vi "Teleop.vi"(10 "Match Info":T1={"Autonomous Elapsed Seconds"=0.0, "TeleOp Elapsed Seconds"=0.0, "Disabled Elapsed Seconds"=0.0, "Visited Autonomous"=FALSE, "Visited TeleOp"=FALSE, "Visited Disabled"=FALSE, "Autonomous Settings"={"Autonomous Style"=enum."Independent", "VI Refnum"=refnum}}, 11 "Call Context":T2) -> ()   [LabVIEW 2020]
doc: "This VI is called for each enabled TeleOp packet received from the DS. It is typically used to read from joysticks and other inputs and update I/O or setpoints for timed control loops. It should complete and return within 20 milliseconds or risk missing DS packets."
uses:
  <vilib>/Rock Robotics/WPI/DriverStation/WPI_DriverStationDerivedRobotMode.ctl
  <vilib>/Rock Robotics/WPI/DriverStation/WPI_DriverStationMatch Info.ctl
  <vilib>/Rock Robotics/WPI/Utilities/WPI_GetSetVariantRefNum.vi
  <vilib>/Rock Robotics/Network Tables/NT Write Boolean Array.vi
  Framework/Robot Global Data.vi
  <vilib>/Rock Robotics/Network Tables/NT Write Variant.vi
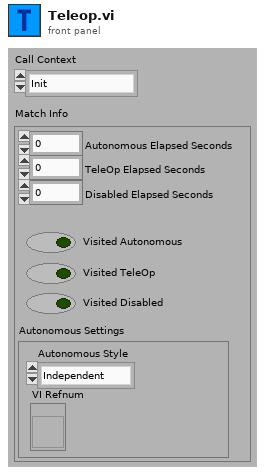
[diagram p1: front panel]
types:
  T1 = typedef "WPI_DriverStationMatch Info.ctl" = cluster{"Autonomous Elapsed Seconds":dbl, "TeleOp Elapsed Seconds":dbl, "Disabled Elapsed Seconds":dbl, "Visited Autonomous":bool, "Visited TeleOp":bool, "Visited Disabled":bool, "Autonomous Settings":cluster{"Autonomous Style":enum16{"Iterative", "Independent"}, "VI Refnum":refnum<vi>}}
  T2 = typedef "WPI_DriverStationDerivedRobotMode.ctl" = enum16{"Init", "Execute", "Stop"}
  T3 = typedef "WPI_JoystickDevRef.ctl" = cluster{"Device":T4}
  T4 = typedef "WPI_JoystickDeviceEnum.ctl" = enum16{"USB 0", "USB 1", "USB 2", "USB 3", "USB 4", "USB 5"}
  T5 = typedef "Command Status Info.ctl" = cluster{"Name":string, "Status":T6, "notifier out":T7}
  T6 = typedef "Completion Status.ctl" = enum16{"Successful", "Aborted", "Incomplete"}
  T7 = typedef "Completion Notifier.ctl" = refnum<notifier>
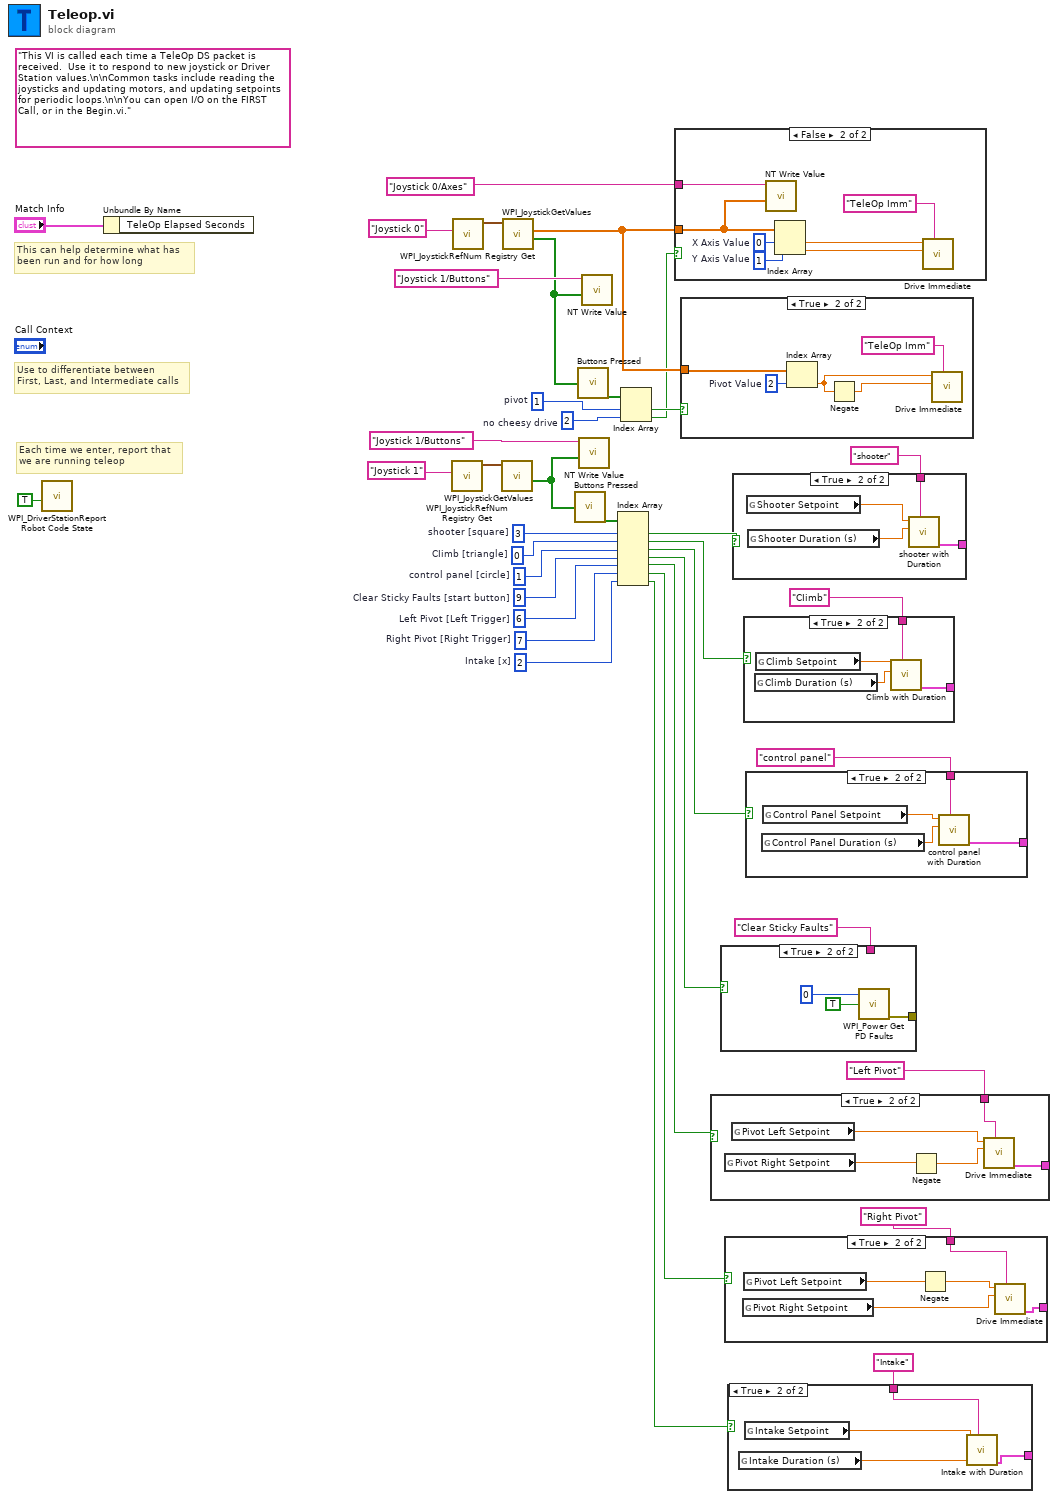
[diagram p0: block diagram]
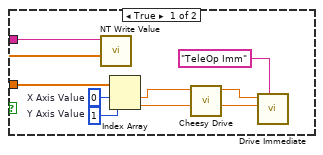
[diagram p2: hidden frame]
diagram:
  w2 = 2  # no cheesy drive
  w7 = 1  # pivot
  w14 = 2  # Intake [x]
  w19 = 7  # Right Pivot [Right Trigger]
  w15 = 6  # Left Pivot [Left Trigger]
  w16 = 9  # Clear Sticky Faults [start button]
  w24 = 1  # control panel [circle]
  w25 = 0  # CIimb [triangle]
  w26 = 3  # shooter [square]
  (unwired) "This VI is called each time a TeleOp DS packet is received.  Use it to respond to new joystick or Driver Station values.\n\nCommon tasks include reading the joysticks and updating motors, and updating setpoints for periodic loops.\n\nYou can open I/O on the FIRST Call, or in the Begin.vi."
  # "Each time we enter, report that\nwe are running teleop"
  # "Use to differentiate between\nFirst, Last, and Intermediate calls"
  # "This can help determine what has\nbeen run and for how long"
  n1 = call <vilib>:"WPI_DriverStationReport Robot Code State.vi"("TeleOp"=TRUE ("Autonomous")) -> ()  [unwired: 10 in, 1 out]
  n2 = Unbundle By Name("Match Info") -> ()  [unwired: 1 out]
  n3 = call <vilib>:"WPI_JoystickRefNum Registry Get.vi"("refnum name"="Joystick 1") -> ("JoystickDevRef"=w11:T3)  [unwired: 1 in, 9 out]
  n4 = call <vilib>:"WPI_JoystickRefNum Registry Get.vi"("refnum name"="Joystick 0") -> ("JoystickDevRef"=w36:T3)  [unwired: 1 in, 9 out]
  n5 = call <vilib>:"WPI_JoystickGetValues.vi"("JoystickDevRef"=w11) -> ("Buttons"=w9:bool[])  [unwired: 6 in, 4 out]
  n6 = call <vilib>:"WPI_JoystickGetValues.vi"("JoystickDevRef"=w36) -> ("Buttons"=w4:bool[], "Axes"=w8:dbl[])  [unwired: 6 in, 3 out]
  n7 = call "Buttons Pressed.vi"("Button Values"=w9) -> ("Button Presses"=w33:bool[])
  n8 = call "Buttons Pressed.vi"("Button Values"=w4) -> ("Button Presses"=w5:bool[])
  n9 = call-poly <vilib>:"NT Write Value.vi"("Boolean Array"=w9, "Name"="Joystick 1/Buttons") -> ()  [unwired: 9 in, 1 out]
  n10 = call-poly <vilib>:"NT Write Value.vi"("Boolean Array"=w4, "Name"="Joystick 1/Buttons") -> ()  [unwired: 9 in, 1 out]
  n11 = Index Array(array=w33, index #1=w26, index #2=w25, index #3=w24, index #4=w16, index #5=w15, index #6=w19, index #7=w14) -> (element #1=w32:bool, element #2=w31:bool, element #3=w27:bool, element #4=w22:bool, element #5=w18:bool, element #6=w17:bool, element #7=w12:bool)
  n12 = Index Array(array=w5, index #1=w7, index #2=w2) -> (element #1=w3:bool, element #2=w1:bool)
  n13 = case shown="False" w1 {
    tunnel: "Joystick 0/Axes" ("Name") -> [w44 w53]
    tunnel: w8 -> [w40 w49]
    frame True {
      w42 = 1  # Y Axis Value
      w43 = 0  # X Axis Value
      n14 = call-poly <vilib>:"NT Write Value.vi"("Variant"=w40, "Name"=w44) -> ()  [unwired: 9 in, 1 out]
      n15 = Index Array(array=w40, index #1=w43, index #2=w42) -> (element #1=w41:dbl, element #2=w45:dbl)
      n16 = call "Cheesy Drive.vi"("Throttle"=w45, "Wheel"=w41) -> ("Right PWM"=w46:dbl, "Left PWM"=w47:dbl)  [unwired: 8 in]
      n17 = call "Drive Immediate.vi"("Description"="TeleOp Imm", "Right Setpoint"=w46, "Left Setpoint"=w47) -> ()  [unwired: 8 in, 1 out]
    }
    frame False {
      w51 = 1  # Y Axis Value
      w52 = 0  # X Axis Value
      n18 = call-poly <vilib>:"NT Write Value.vi"("Variant"=w49, "Name"=w53) -> ()  [unwired: 9 in, 1 out]
      n19 = Index Array(array=w49, index #1=w52, index #2=w51) -> (element #1=w50:dbl, element #2=w54:dbl)
      n20 = call "Drive Immediate.vi"("Description"="TeleOp Imm", "Right Setpoint"=w54, "Left Setpoint"=w50) -> ()  [unwired: 8 in, 1 out]
    }
  }
  n21 = case shown="True" w3 {
    tunnel: w8 -> [_ w58]
    frame False {
    }
    frame True {
      w60 = 2  # Pivot Value
      n22 = Index Array(array=w58, index=w60) -> (element=w57:dbl)
      n23 = Negate(x=w57) -> (-x=w56:dbl)
      n24 = call "Drive Immediate.vi"("Description"="TeleOp Imm", "Right Setpoint"=w56, "Left Setpoint"=w57) -> ()  [unwired: 8 in, 1 out]
    }
  }
  n25 = case shown="True" w18 {
    tunnel: [_ w65] -> _
    tunnel: "Left Pivot" ("Description") -> [_ w64]
    frame False {
    }
    frame True {
      n26 = global read "Robot Global Data.vi" "Pivot Right Setpoint"() -> (w63:dbl)
      n27 = global read "Robot Global Data.vi" "Pivot Left Setpoint"() -> (w62:dbl)
      n28 = Negate(x=w63) -> (-x=w61:dbl)
      n29 = call "Drive Immediate.vi"("Description"=w64, "Right Setpoint"=w61, "Left Setpoint"=w62) -> ("Command Info Out"=w65:T5)  [unwired: 8 in]
    }
  }
  n30 = case shown="True" w22 {
    tunnel: [_ w68] -> _
    tunnel: "Clear Sticky Faults" ("Description") -> [_ _]
    frame False {
    }
    frame True {
      n31 = call <vilib>:"WPI_Power Get PD Faults.vi"("Power Distribution (def)"=u8 0, "Clear Sticky Faults"=TRUE) -> ("error out"=w68:errorcluster)  [unwired: 10 in, 3 out]
    }
  }
  n32 = case shown="True" w17 {
    tunnel: [_ w73] -> _
    tunnel: "Right Pivot" ("Description") -> [_ w72]
    frame False {
    }
    frame True {
      n33 = global read "Robot Global Data.vi" "Pivot Right Setpoint"() -> (w69:dbl)
      n34 = global read "Robot Global Data.vi" "Pivot Left Setpoint"() -> (w70:dbl)
      n35 = Negate(x=w70) -> (-x=w71:dbl)
      n36 = call "Drive Immediate.vi"("Description"=w72, "Right Setpoint"=w69, "Left Setpoint"=w71) -> ("Command Info Out"=w73:T5)  [unwired: 8 in]
    }
  }
  n37 = case shown="True" w12 {
    tunnel: [_ w77] -> _
    tunnel: "Intake" ("Description") -> [_ w76]
    frame False {
    }
    frame True {
      n38 = global read "Robot Global Data.vi" "Intake Duration (s)"() -> (w74:dbl)
      n39 = global read "Robot Global Data.vi" "Intake Setpoint"() -> (w75:dbl)
      n40 = call "Intake with Duration .vi"("Description"=w76, "Duration (s)"=w74, "Setpoint"=w75) -> ("Command Info Out"=w77:T5)  [unwired: 8 in]
    }
  }
  n41 = case shown="True" w32 {
    tunnel: [_ w81] -> _
    tunnel: "shooter" ("Description") -> [_ w80]
    frame False {
    }
    frame True {
      n42 = global read "Robot Global Data.vi" "Shooter Setpoint"() -> (w79:dbl)
      n43 = global read "Robot Global Data.vi" "Shooter Duration (s)"() -> (w78:dbl)
      n44 = call "shooter with Duration .vi"("Description"=w80, "Duration (s)"=w78, "Setpoint"=w79) -> ("Command Info Out"=w81:T5)  [unwired: 8 in]
    }
  }
  n45 = case shown="True" w31 {
    tunnel: [_ w85] -> _
    tunnel: "CIimb" ("Description") -> [_ w84]
    frame False {
    }
    frame True {
      n46 = global read "Robot Global Data.vi" "Climb Duration (s)"() -> (w82:dbl)
      n47 = global read "Robot Global Data.vi" "Climb Setpoint"() -> (w83:dbl)
      n48 = call "CIimb with Duration.vi"("Description"=w84, "Duration (s)"=w82, "Setpoint"=w83) -> ("Command Info Out"=w85:T5)  [unwired: 8 in]
    }
  }
  n49 = case shown="True" w27 {
    tunnel: [_ w89] -> _
    tunnel: "control panel" ("Description") -> [_ w88]
    frame False {
    }
    frame True {
      n50 = global read "Robot Global Data.vi" "Control Panel Duration (s)"() -> (w86:dbl)
      n51 = global read "Robot Global Data.vi" "Control Panel Setpoint"() -> (w87:dbl)
      n52 = call "control panel with Duration.vi"("Description"=w88, "Duration (s)"=w86, "Setpoint"=w87) -> ("Command Info Out"=w89:T5)  [unwired: 8 in]
    }
  }
